vi "Build Sections Document.vi"(8 "error in":errorcluster, 11 "Targets":T1[](array[typedef])) -> (0 "error out":errorcluster, 3 "Sections":refnum<class "Section.lvclass">[](array[class]))   [LabVIEW 2021, in "TAF Proj Document Type.lvlib" / "TAF Proj.lvclass"]
uses:
  <vilib>/Wovalab/AntiDoc/Document Type/Add-ons/LabVIEW TAF Project/TAF Proj/TAF Proj.lvclass
  <vilib>/Wovalab/AntiDoc/Section/Section.lvclass
  <vilib>/Wovalab/AntiDoc/Document Type/Add-ons/LabVIEW TAF Project/Project Parser/Target--cluster.ctl
  <vilib>/Wovalab/AntiDoc/Document Type/Add-ons/LabVIEW TAF Project/Custom Errors/Custom Errors.lvclass
  <vilib>/Wovalab/AntiDoc/Document Type/Add-ons/LabVIEW TAF Project/Classes Overview/Classes Overview.lvclass
  <vilib>/Wovalab/AntiDoc/Document Type/Add-ons/LabVIEW TAF Project/Dqmh Modules Overview/Dqmh Modules Overview.lvclass
  <vilib>/Wovalab/AntiDoc/Document Type/Add-ons/LabVIEW TAF Project/FrontPanelGUI/FrontPanelGUI.lvclass
  <vilib>/Wovalab/AntiDoc/Document Type/Add-ons/LabVIEW TAF Project/Project Parser/Blocs--cluster.ctl
  <vilib>/Wovalab/AntiDoc/Document Type/Add-ons/LabVIEW TAF Project/Dqmh Module/Dqmh Module.lvclass
  <vilib>/Wovalab/AntiDoc/Document Type/Add-ons/LabVIEW TAF Project/Class/Class.lvclass
  <vilib>/Wovalab/AntiDoc/Document Type/Add-ons/LabVIEW TAF Project/Lib/Lib.lvclass
  <vilib>/Wovalab/AntiDoc/Document Type/Add-ons/LabVIEW TAF Project/TAFConfiguration/TAFConfiguration.lvclass
  <vilib>/Wovalab/AntiDoc/Sub Section/Sub Section.lvclass
  C:/Program Files (x86)/National Instruments/LabVIEW 2021/vi.lib/Wovalab/AntiDoc/Section/Section.lvclass
  <vilib>/Wovalab/AntiDoc/Progress Bar/Progress Bar.lvlib
  <vilib>/Wovalab/AntiDoc/Document Type/Add-ons/LabVIEW TAF Project/Project Parser/Project Parser.lvlib
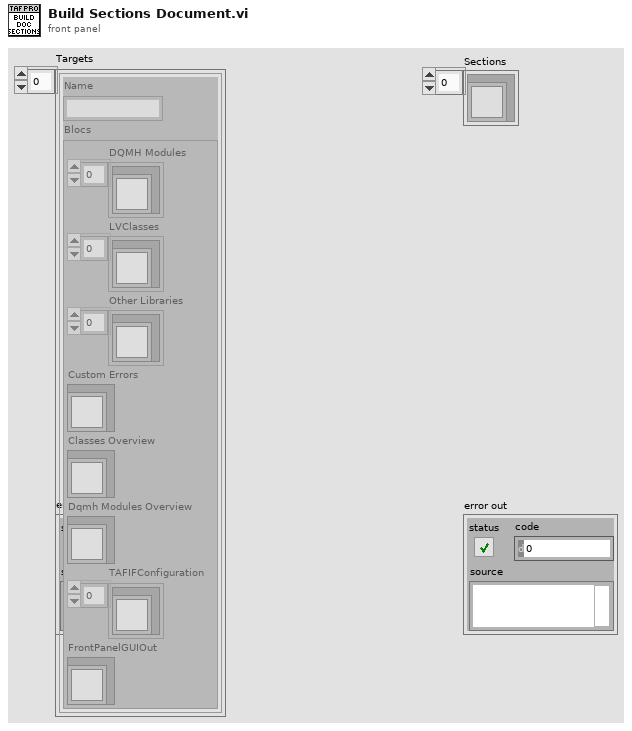
[diagram p1: front panel]
types:
  T1 = typedef "TAF Proj Document Type.lvlib/Project Parser.lvlib/Target--cluster.ctl" = cluster{"Name":string, "Blocs":T2}
  T2 = typedef "TAF Proj Document Type.lvlib/Project Parser.lvlib/Blocs--cluster.ctl" = cluster{"DQMH Modules":refnum<class "Dqmh Module.lvclass">[], "LVClasses":refnum<class "Class.lvclass">[], "Other Libraries":refnum<class "Lib.lvclass">[], "Custom Errors":refnum<class "Custom Errors.lvclass">, "Classes Overview":refnum<class "Classes Overview.lvclass">, "Dqmh Modules Overview":refnum<class "Dqmh Modules Overview.lvclass">, "TAFIFConfiguration":refnum<class "TAFConfiguration.lvclass">[], "FrontPanelGUIOut":refnum<class "FrontPanelGUI.lvclass">}
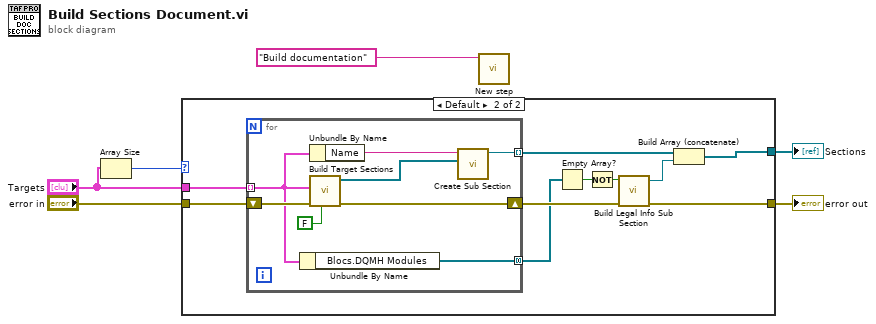
[diagram p0: block diagram]
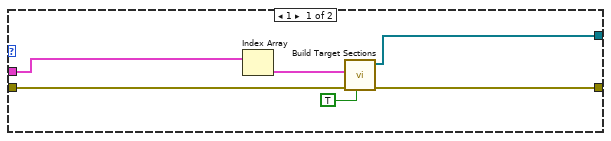
[diagram p2: hidden frame]
diagram:
  n1 = Array Size(array="Targets") -> (size(s)=w2:i32)
  n2 = case shown="Default" w2 {
    tunnel: [w12 w20] -> w6
    tunnel: "error in" -> [w11 w22]
    tunnel: [w8 w14] -> w4
    tunnel: "Targets" -> [w10 w19]
    frame 1 {
      n3 = Index Array(array=w10) -> (element=w9:T1)  [unwired: 1 in]
      n4 = call <vilib>:"Build Target Sections.vi"("Add Legal Section"=TRUE, "error in"=w11, "Target"=w9) -> ("error out"=w12:errorcluster, "Target Sections"=w8:refnum<class "Section.lvclass">[])  [unwired: 7 in]
    }
    frame Default {
      n5 = for {
        tunnel: [w25] -> w13 mode=indexing
        tunnel: w19 -> [w27] mode=indexing
        shift-right: [w29] -> w21
        shift-left: w22 -> [w30]
        tunnel: [w28] -> w16 mode=concatenating
        n6 = Unbundle By Name(w27) -> ("Blocs.DQMH Modules"=w28:refnum<class "Dqmh Module.lvclass">[])
        n7 = Unbundle By Name(w27) -> ("Name"=w24:string)
        n8 = call <vilib>:"Build Target Sections.vi"("Add Legal Section"=FALSE, "error in"=w30, "Target"=w27) -> ("error out"=w29:errorcluster, "Target Sections"=w23:refnum<class "Section.lvclass">[])  [unwired: 7 in]
        n9 = call <vilib>:"Create Sub Section.vi"("Sections"=w23, "Name"=w24) -> ("Sub Section out"=w25:refnum<class "Sub Section.lvclass">)  [unwired: 8 in, 1 out]
      }
      n10 = Empty Array?(array=w16) -> (empty?=w17:bool)
      n11 = Not(x=w17) -> (.not. x?=w18:bool)
      n12 = call <vilib>:"Build Legal Info Sub Section.vi"("error in"=w21, "Has DQMH modules"=w18) -> ("error out"=w20:errorcluster, "Lv Proj Document Type:TAF Proj"=w15:refnum<class "Sub Section.lvclass">)  [unwired: 8 in]
      n13 = Build Array (concatenate)(w13, w15) -> (w14:refnum<class "Sub Section.lvclass">[])
    }
  }
  "error out" <- w6
  "Sections" <- w4
  n14 = call <vilib>:"New step.vi"("Description"="Build documentation") -> ()  [unwired: 10 in, 1 out]
